vi "19.6-DirectIIR-4th Order.vi"() -> ()   [LabVIEW 2020]
doc: "Uses the Median Filter VI to analyze pulses in the presence of noise. The example generates a pulse contaminated with Gaussian noise and applies a median filter. For comparison purposes, the VI computes the pulse parameters of the filtered pulse."
uses:
  <vilib>/Analysis/3filter.llb/IIR Filter (DBL).vi
  <vilib>/Analysis/NI_AALBase.lvlib
panel:
  in  "stop":bool
  out "Sig":dbl[](graph)
  in  "Fc":dbl(slide)=299.22077922077926 step=1.0 scale=0.0..512.0 scale format="%#_2f"
  out "Filtered1":dbl[](graph)
  out "H[k]1":dbl[](graph)
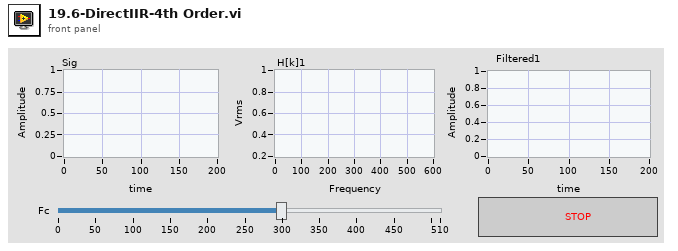
[diagram p1: front panel]
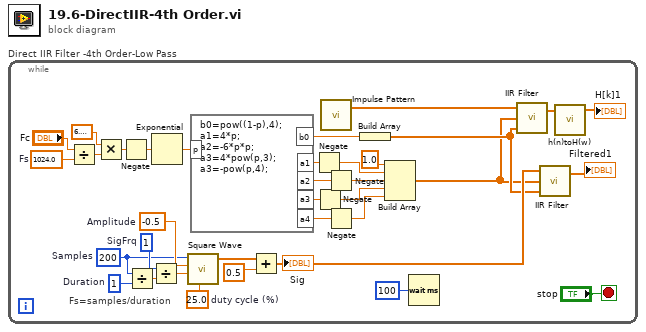
[diagram p0: block diagram]
diagram:
  n1 = while "Direct IIR Filter -4th Order-Low Pass" {
    stop <- "stop" stop-if-true
    w9 = 1024.0  # Fs
    w26 = 1  # Duration
    w33 = 1  # SigFrq
    w34 = 25.0  # duty cycle (%)
    w35 = -0.5  # Amplitude
    w28 = 200  # Samples
    # "Fs=samples/duration"
    n2 = Divide(x="Fc", y=w9) -> (x/y=w14:dbl)
    n3 = Multiply(x=6.283185307179586, y=w14) -> (x*y=w12:dbl)
    n4 = Negate(x=w12) -> (-x=w13:dbl)
    n5 = Divide(x=w28, y=w26) -> (x/y=w27:dbl)
    n6 = Divide(x=w33, y=w27) -> (x/y=w30:dbl)
    n7 = Exponential(1:w13) -> (0:w8:dbl)
    n8 = call <vilib>:"Square Wave.vi"("samples"=w28, "amplitude"=w35, "frequency"=w30, "duty cycle (%)"=w34) -> ("square wave"=w32:dbl[])  [unwired: 2 in, 2 out]
    n9 = formula code="b0=pow((1-p),4);\na1=4*p;\na2=-6*p*p;\na3=4*pow(p,3);\na3=-pow(p,4);"("p"=w8) -> ("b0"=w21:dbl, "a1"=w23:dbl, "a2"=w22:dbl, "a3"=w6:dbl, "a4"=w7:dbl)
    n10 = Add(x=w32, y=0.5) -> (x+y=w20:dbl[])
    "Sig" <- w20
    n11 = Negate(x=w23) -> (-x=w18:dbl)
    n12 = Negate(x=w6) -> (-x=w4:dbl)
    n13 = call <vilib>:"Impulse Pattern.vi"() -> ("Impulse Pattern"=w2:dbl[])  [unwired: 3 in, 1 out]
    n14 = Negate(x=w22) -> (-x=w17:dbl)
    n15 = Negate(x=w7) -> (-x=w5:dbl)
    n16 = Build Array(w21) -> (w15:dbl[])
    n17 = Build Array(1.0 ("element"), w18, w17, w4, w5) -> (w3:dbl[])
    n18 = Wait (ms)(milliseconds to wait=u32 100) -> ()  [unwired: 1 out]
    n19 = call-poly <vilib>:"IIR Filter.vi"("Forward Coefficients"=w15, "Reverse Coefficients"=w3, "X"=w2) -> ("Filtered X"=w29:dbl[])  [unwired: 1 in, 1 out]
    n20 = call-poly <vilib>:"IIR Filter.vi"("Forward Coefficients"=w15, "Reverse Coefficients"=w3, "X"=w20) -> ("Filtered X"=→"Filtered1":dbl[])  [unwired: 1 in, 1 out]
    n21 = call "h(n)toH(w).vi"("h(n)"=w29) -> ("Mag H(w)"=→"H[k]1":dbl[])  [unwired: 1 in, 2 out]
  }
